vi "ex7-8.vi"() -> ()   [LabVIEW 2013]
panel:
  out "size(s)":i32
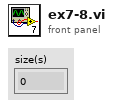
[diagram p1: front panel]
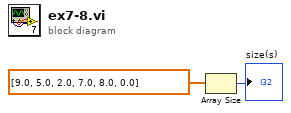
[diagram p0: block diagram]
diagram:
  n1 = Array Size(array=dbl[] [9.0, 5.0, 2.0, 7.0, 8.0, 0.0]) -> (size(s)=→"size(s)":i32)
